vi "Blocking Read Response.vi"(8 "error in (no error)":errorcluster, 9 "Responses in":T1[](array[typedef]) {"Command" items=["Constant Speed Tracking"=8, "Echo"=55, "Error"=255, "Home"=1, "Limit Active"=9, "Manual Move Tracking"=10, "Move Absolute"=20, "Move at Constant Speed"=22, "Move Relative"=21, "Renumber"=2, "Restore Settings"=36, "Stop"=23]}, 11 "VISA resource name":refnum<visa-resource-name>) -> (0 "error out":errorcluster, 1 "Responses out":T1[](array[typedef]) {"Command" items=["Constant Speed Tracking"=8, "Echo"=55, "Error"=255, "Home"=1, "Limit Active"=9, "Manual Move Tracking"=10, "Move Absolute"=20, "Move at Constant Speed"=22, "Move Relative"=21, "Renumber"=2, "Restore Settings"=36, "Stop"=23]}, 2 "Response":T1 {"Command" items=["Constant Speed Tracking"=8, "Echo"=55, "Error"=255, "Home"=1, "Limit Active"=9, "Manual Move Tracking"=10, "Move Absolute"=20, "Move at Constant Speed"=22, "Move Relative"=21, "Renumber"=2, "Restore Settings"=36, "Stop"=23]}, 3 "VISA resource name out":refnum<visa-resource-name>)   [LabVIEW 2020, in "ZaberTSeries.lvlib"]
doc: "Reads a response packet from the serial port. If no response is waiting, this blocks until a response is received. See Read.vi for one that doesn't block."
uses:
  ZaberTSeries.lvlib
  Utility/Response.ctl
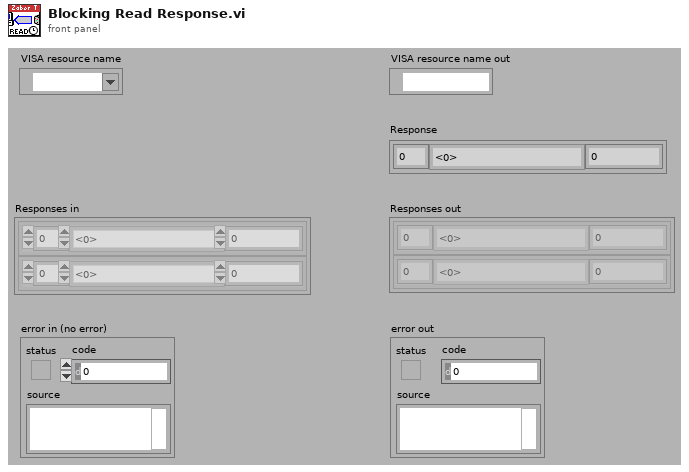
[diagram p1: front panel]
types:
  T1 = typedef "ZaberTSeries.lvlib/Response.ctl" = cluster{"Device Number":u8, "Command":u8, "Data":i32}
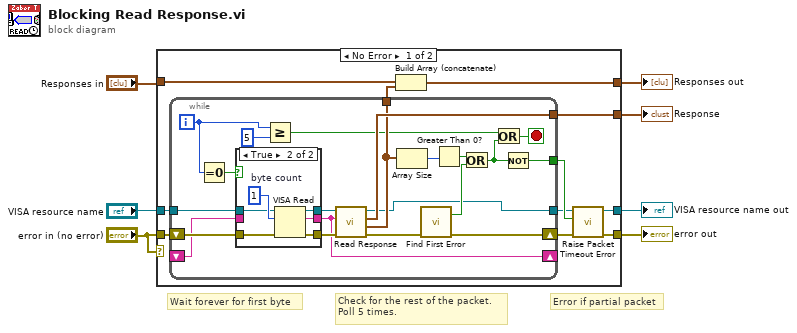
[diagram p0: block diagram]
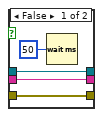
[diagram p2: hidden frame]
diagram:
  # "Error if partial packet"
  # "Check for the rest of the packet.\nPoll 5 times."
  # "Wait forever for first byte"
  n1 = case shown="No Error" "error in (no error)" {
    tunnel: "VISA resource name" -> [w10 w51]
    tunnel: "error in (no error)" -> [w9 w50]
    tunnel: [w13 w50] -> w6
    tunnel: [w8 w51] -> w5
    tunnel: "Responses in" -> [w18 w52]
    tunnel: [w16 _] -> w3
    tunnel: [w17 w52] -> w2
    frame No Error {
      n2 = while {
        shift-right: [w38] -> w14
        shift-left: w9 -> [w31]
        tunnel: [w37] -> w16
        tunnel: [w21] -> w15
        tunnel: [w34] -> w12
        tunnel: w10 -> [w32]
        tunnel: [w25] -> w11
        shift-right: [w19] -> _
        shift-left: _ -> [w20]
        i -> [w28]
        stop <- w24 stop-if-true
        n3 = Equal To 0?(x=w28) -> (x = 0?=w33:bool)
        n4 = case shown="True" w33 {
          tunnel: w32 -> [w42 w48]
          tunnel: w31 -> [w41 w47]
          tunnel: [w41 w46] -> w30
          tunnel: [w42 w45] -> w29
          tunnel: [w40 w44] -> w19
          tunnel: w20 -> [w40 _]
          frame False {
            n5 = Wait (ms)(milliseconds to wait=u32 50) -> ()  [unwired: 1 out]
          }
          frame True {
            w49 = u32 1  # byte count
            n6 = VISA Read(VISA resource name=w48, byte count=w49, error in (no error)=w47) -> (VISA resource name out=w45:refnum<visa-resource-name>, read buffer=w44:string, error out=w46:errorcluster)  [unwired: 1 out]
          }
        }
        n7 = Greater Or Equal?(x=w28, y=5) -> (x >= y?=w22:bool)
        n8 = call "Read Response.vi"("error in (no error)"=w30, "Partial Packet"=w19, "VISA resource name"=w29) -> ("error out"=w26:errorcluster, "Responses out"=w34:T1[], "Response"=w37:T1, "VISA resource name out"=w25:refnum<visa-resource-name>)  [unwired: 4 in, 1 out]
        n9 = Array Size(array=w34) -> (size(s)=w39:i32)
        n10 = call <vilib>:"Find First Error.vi"("error in (no error)"=w26) -> ("error out"=w38:errorcluster, "error?"=w36:bool)  [unwired: 3 in]
        n11 = Greater Than 0?(x=w39) -> (x > 0?=w35:bool)
        n12 = Or(x=w35, y=w36) -> (x .or. y?=w23:bool)
        n13 = Or(x=w22, y=w23) -> (x .or. y?=w24:bool)
        n14 = Not(x=w23) -> (.not. x?=w21:bool)
      }
      n15 = Build Array (concatenate)(w18, w12) -> (w17:T1[])
      n16 = call "Raise Packet Timeout Error.vi"("error in (no error)"=w14, "Enable Packet Timeout Error"=w15, "VISA resource name"=w11) -> ("error out"=w13:errorcluster, "VISA resource name out"=w8:refnum<visa-resource-name>)  [unwired: 7 in]
    }
    frame Error {
    }
  }
  "error out" <- w6
  "Response" <- w3
  "VISA resource name out" <- w5
  "Responses out" <- w2
